vi "init.vi"(8 "error in (no error)":errorcluster, 11 "simulado in":refnum<class "simulado.lvclass">) -> (0 "error out":errorcluster, 3 "simulado out":refnum<class "simulado.lvclass">)   [LabVIEW 2019, in "simulado.lvclass"]
uses:
  simulado.lvclass
  simulado.lvclass/simulado.ctl
panel:
  in  "device":string
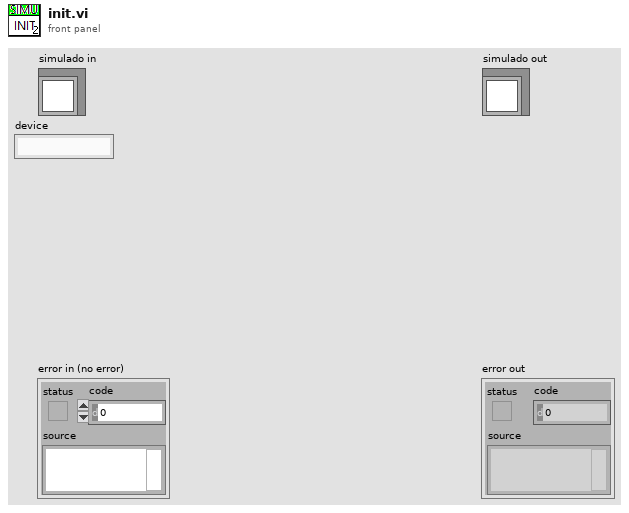
[diagram p1: front panel]
types:
  T1 = enum16{"get parameter", "Set parameters", "reset parameter", ""}
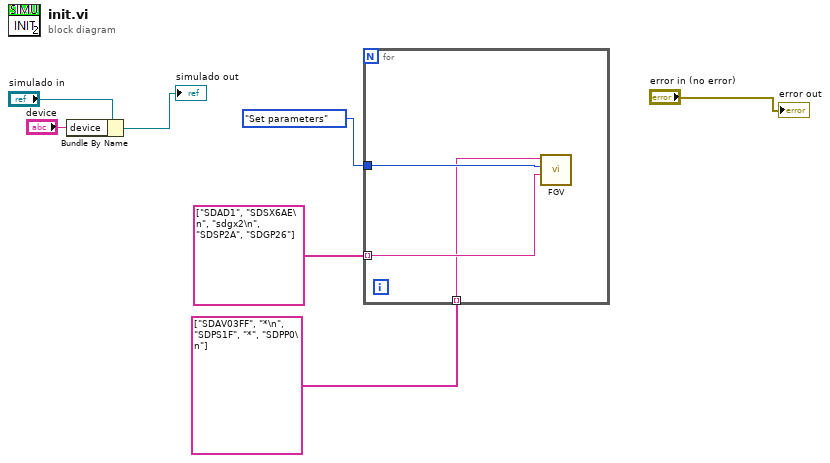
[diagram p0: block diagram]
diagram:
  n1 = Bundle By Name(cluster="simulado in", "device"="device") -> (→"simulado out":refnum<class "simulado.lvclass">)
  n2 = for {
    tunnel: T1."Set parameters" ("functions") -> [w10]
    tunnel: string[] ["SDAD1", "SDSX6AE\n", "sdgx2\n", "SDSP2A", "SDGP26"] ("command") -> [w9] mode=indexing
    tunnel: string[] ["SDAV03FF", "*\n", "SDPS1F", "*", "SDPP0\n"] ("command") -> [w8] mode=indexing
    n3 = call "FGV.vi"("command"=w9, "functions"=w10, "response to save"=w8) -> ()  [unwired: 7 in, 2 out]
  }
  "error out" <- "error in (no error)"
